vi "Receiver_Example.vi"() -> ()   [LabVIEW 2014]
panel:
  in  "downsampling factor":i32
  out "created new?":bool
  out "string 2":string
  in  "stop":bool
  out "USRP CoercedParamters":T1={"coerced IQ rate"=100000.0, "coerced carrier frequency"=100000.0, "coerced gain"=0.0} {"coerced gain" format="%#_6f"; "coerced carrier frequency" format="%#_6p"; "coerced IQ rate" format="%#_6p"}
  out "error out":errorcluster
  in  "Trigger level":dbl=0.005 format="%f"
  in  "error in (no error)":errorcluster
  in  "USRP ControledParameters":T2={"active antenna"="RX2", "gain"=20.0, "carrier frequency"=5800000000.0, "IQ rate"=2000000.0} {"IQ rate" format="%#_6p"; "carrier frequency" format="%#_6p"; "gain" format="%#_6f"}
  in  "device names":refnum<k15>="NI2900"
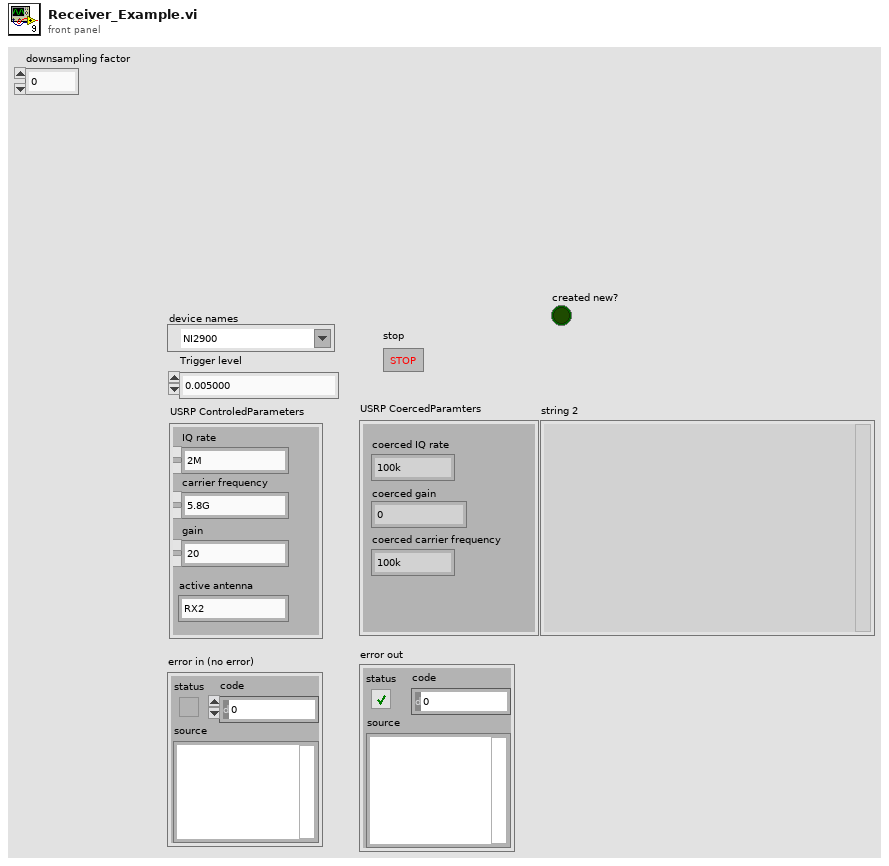
[diagram p1: front panel]
types:
  T1 = cluster{"coerced IQ rate":dbl, "coerced carrier frequency":dbl, "coerced gain":dbl}
  T2 = cluster{"active antenna":string, "gain":dbl, "carrier frequency":dbl, "IQ rate":dbl}
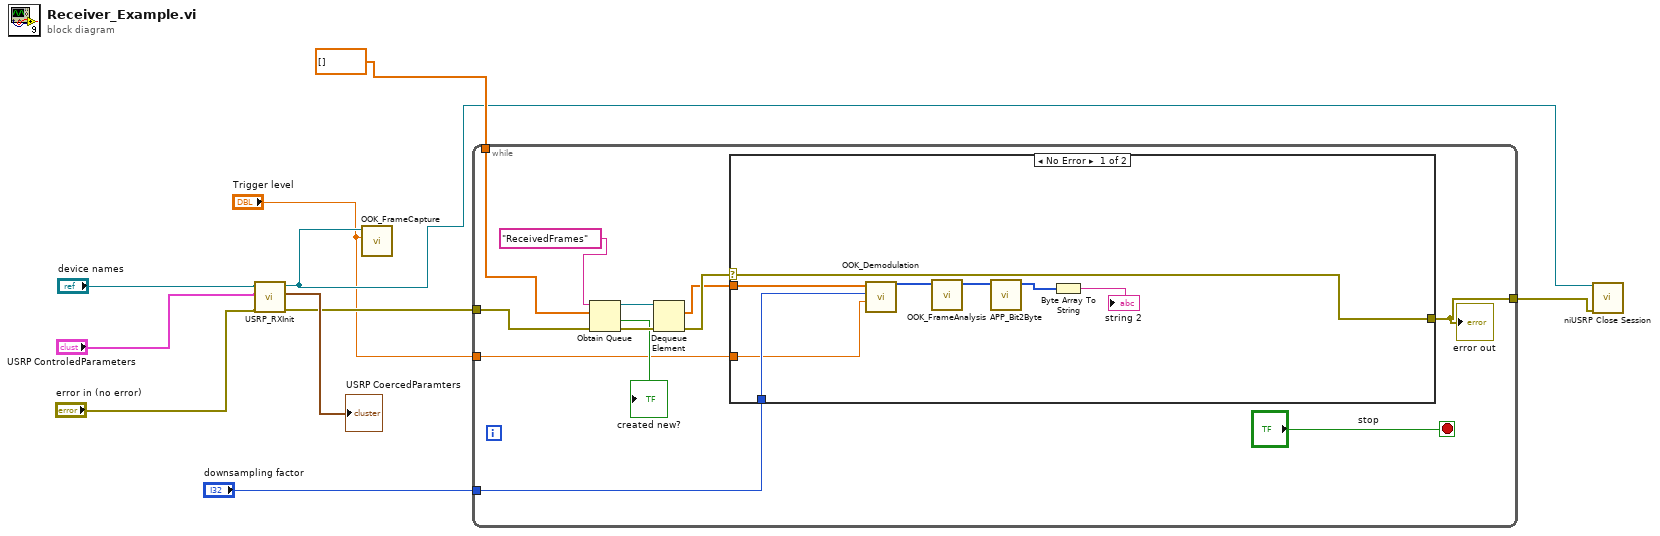
[diagram p0: block diagram]
diagram:
  n1 = call "USRP_RXInit.vi"("device names"="device names", "USRP ControledParameters"="USRP ControledParameters", "error in (no error)"="error in (no error)") -> ("session handle out"=w3:refnum<k15>, "USRP CoercedParamters"=→"USRP CoercedParamters":T1, "error out"=w6:errorcluster)  [unwired: 5 in]
  n2 = call "OOK_FrameCapture.vi"("Trigger level"="Trigger level", "session handle"=w3) -> ()  [unwired: 9 in]
  n3 = while {
    tunnel: w6 -> [w20]
    tunnel: cdb[] [] -> [w21]
    tunnel: [w13] -> w5
    tunnel: "downsampling factor" -> [w12]
    tunnel: "Trigger level" -> [w11]
    stop <- "stop" stop-if-true
    n4 = Obtain Queue(name (unnamed)="ReceivedFrames", element data type=w21, error in (no error)=w20) -> (queue out=w19:refnum<queue>, created new?=→"created new?":bool, error out=w16:errorcluster)  [unwired: 2 in]
    n5 = Dequeue Element(queue=w19, error in (no error)=w16) -> (element=w17:cdb[], error out=w18:errorcluster)  [unwired: 1 in, 2 out]
    n6 = case shown="No Error" w18 {
      selector: w18 -> [w25 w31]
      tunnel: w17 -> [w30 _]
      tunnel: [w25 w31] -> w13
      tunnel: w12 -> [w29 _]
      tunnel: w11 -> [w28 _]
      frame No Error {
        n7 = call "OOK_Demodulation.vi"("trigger level"=w28, "downsampling factor"=w29, "input symbol stream"=w30) -> ("output bit stream"=w24:i8[])  [unwired: 8 in]
        n8 = call "OOK_FrameAnalysis.vi"("input bit stream"=w24) -> ("data bit stream"=w23:i8[])  [unwired: 10 in]
        n9 = call "APP_Bit2Byte.vi"("input bit stream"=w23) -> ("output byte stream"=w27:u8[])  [unwired: 10 in]
        n10 = Byte Array To String(unsigned byte array=w27) -> (string=→"string 2":string)
      }
      frame Error {
      }
    }
    "error out" <- w13
  }
  n11 = call <instrlib>:"niUSRP Close Session.vi"("session handle"=w3, "error in (no error)"=w5) -> ()  [unwired: 13 in, 1 out]
